vi "Configure Application Log.vi"(4 "Configuration.Level":T1=enum."Debug", 6 "Configuration.Enabled":bool=TRUE, 7 "Configuration.Call Chain":bool, 8 "error in (no error)":errorcluster, 11 "Application Log in":refnum<class "Application Log.lvclass">) -> (0 "error out":errorcluster, 3 "Application Log out":refnum<class "Application Log.lvclass">)   [LabVIEW 2016, in "Stream Log.lvlib" / "Application Log.lvclass"]
doc: "--\nCopyright © 2017 Composed SystemsI All rights reserved.\n\nAuthor: Jon McBee <jon.mcbee@composed.io>\n\nThis library is provided \"AS IS\" ,WITHOUT WARRANTIES OR\nCONDITIONS OF ANY KIND, either express or implied.\n\nComposed Systems -- composed.io\n\nStream 0.0.1.1\nJon McBee - Composed Systems\nCopyright (c) 2017, Composed Systems"
uses:
  <userlib>/Composed Systems/Stream/Log/Application Log/Application Log.lvclass
  <userlib>/Composed Systems/Stream/Log/Application Log/Log Level.ctl
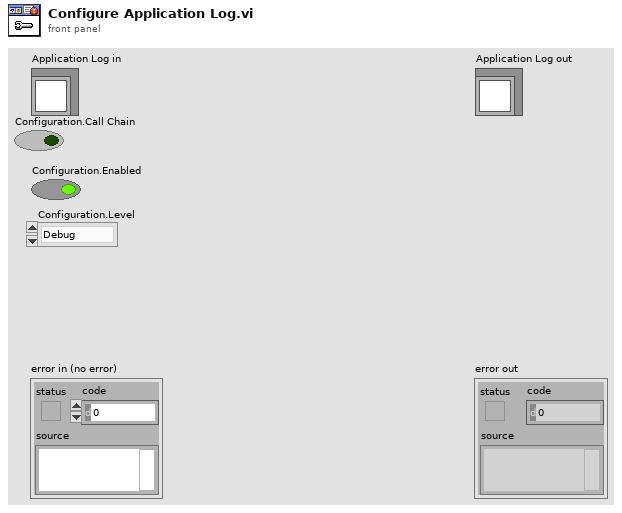
[diagram p1: front panel]
types:
  T1 = typedef "Stream Log.lvlib/Application Log.lvclass/Log Level.ctl" = enum16{"Imperative", "Major", "Minor", "Debug", "Off"}
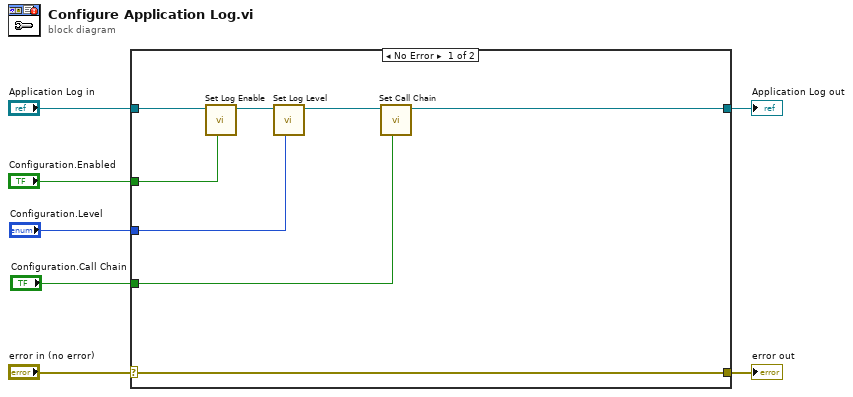
[diagram p0: block diagram]
diagram:
  n1 = case shown="No Error" "error in (no error)" {
    selector: "error in (no error)" -> [w15 w17]
    tunnel: [w15 w17] -> w6
    tunnel: [w9 w16] -> w4
    tunnel: "Application Log in" -> [w13 w16]
    tunnel: "Configuration.Enabled" -> [w12 _]
    tunnel: "Configuration.Level" -> [w11 _]
    tunnel: "Configuration.Call Chain" -> [w8 _]
    frame No Error {
      n2 = call <userlib>:"Set Log Enable.vi"("Configuration.Enabled"=w12, "Application Log in"=w13) -> ("Application Log out"=w14:refnum<class "Application Log.lvclass">)  [unwired: 8 in, 1 out]
      n3 = call <userlib>:"Set Log Level.vi"("Configuration.Level"=w11, "Application Log in"=w14) -> ("Application Log out"=w10:refnum<class "Application Log.lvclass">)  [unwired: 8 in, 1 out]
      n4 = call <userlib>:"Set Call Chain.vi"("Configuration.Call Chain"=w8, "Application Log in"=w10) -> ("Application Log out"=w9:refnum<class "Application Log.lvclass">)  [unwired: 8 in, 1 out]
    }
    frame Error {
    }
  }
  "error out" <- w6
  "Application Log out" <- w4
